vi "Init.vi"(8 "error in (no error)":errorcluster caption="错误输入（无错误）", 11 "同事（抽象） 输入":refnum<class "Colleague.lvclass"> caption="DNL_LabVIEW Object in") -> (0 "error out":errorcluster caption="错误输出", 3 "同事（抽象） 输出":refnum<class "Colleague.lvclass"> caption="DNL_LabVIEW Object out")   [LabVIEW 2011, in "Colleague.lvclass"]
uses:
  Colleague.lvclass
  Colleague.lvclass/Colleague.ctl
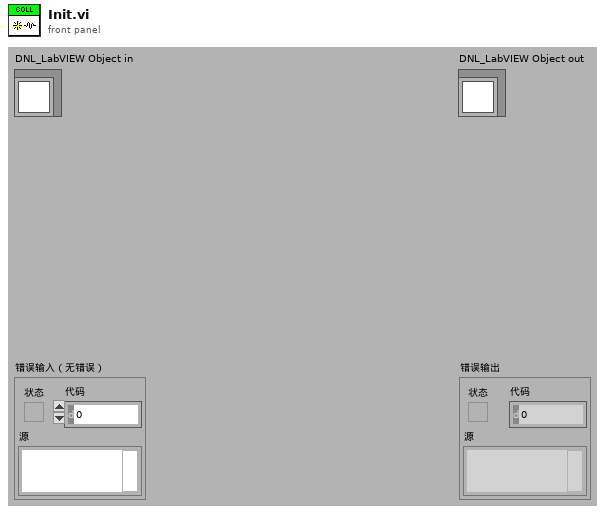
[diagram p1: front panel]
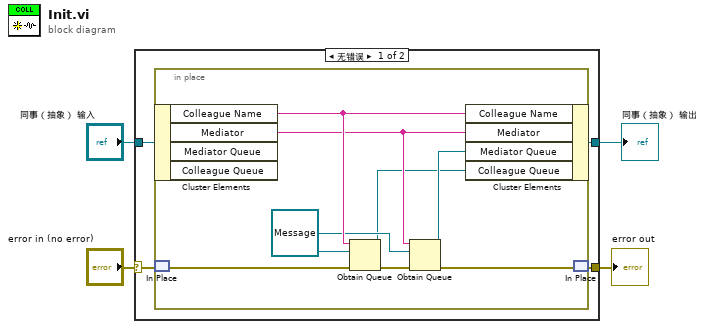
[diagram p0: block diagram]
diagram:
  n1 = case shown="无错误" "error in (no error)" {
    selector: "error in (no error)" -> [w7 w18]
    tunnel: [w6 w18] -> w3
    tunnel: [w5 w17] -> w1
    tunnel: "同事（抽象） 输入" -> [w8 w17]
    frame No Error {
      n2 = in-place {
        w11 = refnum<class "Message.lvclass"> refnum ("Message.lvclass")
        n3 = in-place-cluster #1(w8) -> ("Colleague Name"=w13:string, "Mediator"=w12:string)  [unwired: 2 out]
        n4 = in-place-match #2(w7) -> (w16:errorcluster)
        n5 = Obtain Queue(name (unnamed)=w13, element data type=w11, error in (no error)=w16) -> (queue out=w9:refnum<queue>, error out=w15:errorcluster)  [unwired: 2 in, 1 out]
        n6 = Obtain Queue(name (unnamed)=w12, element data type=w11, error in (no error)=w15) -> (queue out=w10:refnum<queue>, error out=w14:errorcluster)  [unwired: 2 in, 1 out]
        n7 = in-place-cluster #1("Colleague Name"=w13, "Mediator"=w12, "Mediator Queue"=w10, "Colleague Queue"=w9) -> (w5:refnum<class "Colleague.lvclass">)
        n8 = in-place-match #2(w14) -> (w6:errorcluster)
      }
    }
    frame Error {
    }
  }
  "error out" <- w3
  "同事（抽象） 输出" <- w1
